vi "Main.vi"() -> ()   [LabVIEW 2018]
panel:
  out "Result":dbl
  in  "Operation":enum16{"Add", "Subtract", "Multiply", "Divide"}(ring)
  in  "Number 2":dbl
  in  "Number 1":dbl
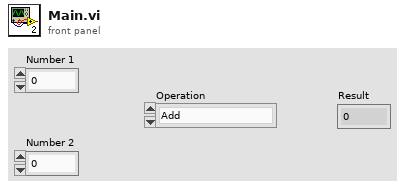
[diagram p1: front panel]
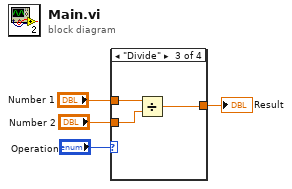
[diagram p0: block diagram]
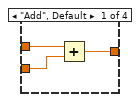
[diagram p2: hidden frame]
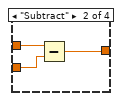
[diagram p3: hidden frame]
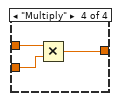
[diagram p4: hidden frame]
diagram:
  n1 = case shown="\"Divide\"" "Operation" {
    tunnel: "Number 1" -> [w7 w10 w13 w16]
    tunnel: "Number 2" -> [w6 w9 w12 w15]
    tunnel: [w5 w8 w11 w14] -> w1
    frame "Add", Default {
      n2 = Add(x=w7, y=w6) -> (x+y=w5:dbl)
    }
    frame "Subtract" {
      n3 = Subtract(x=w10, y=w9) -> (x-y=w8:dbl)
    }
    frame "Divide" {
      n4 = Divide(x=w13, y=w12) -> (x/y=w11:dbl)
    }
    frame "Multiply" {
      n5 = Multiply(x=w16, y=w15) -> (x*y=w14:dbl)
    }
  }
  "Result" <- w1
